vi "Initialise.vi"(8 "error in (no error)":errorcluster, 11 "Max Steps (100)":i32=3) -> (0 "error out":errorcluster, 3 "Sequencer out":refnum<class "Sequencer.lvclass">)   [LabVIEW 2015, in "Sequencer.lvclass"]
uses:
  Sequencer.lvclass
  Single Step Data.ctl
  Messaging/Message/Message.lvclass
  Sequencer.lvclass/Sequencer.ctl
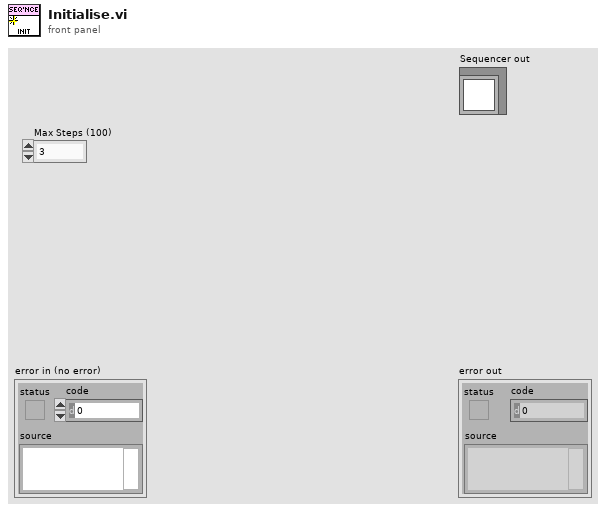
[diagram p1: front panel]
types:
  T1 = typedef "Sequencer.lvclass/Single Step Data.ctl" = cluster{"Step":string, "Parameter":variant, "Reply Channel":refnum<notifier>}
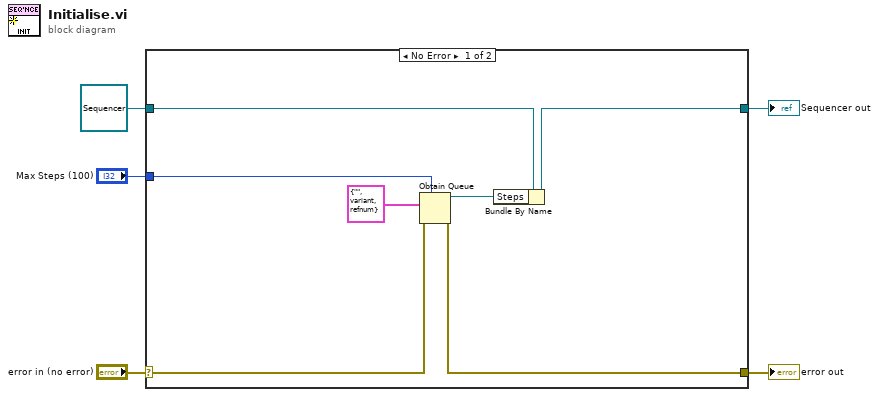
[diagram p0: block diagram]
diagram:
  n1 = case shown="No Error" "error in (no error)" {
    selector: "error in (no error)" -> [w7 w14]
    tunnel: [w6 w14] -> w4
    tunnel: [w8 w13] -> w2
    tunnel: refnum<class "Sequencer.lvclass"> refnum ("Sequencer in") -> [w10 w13]
    tunnel: "Max Steps (100)" -> [w11 _]
    frame No Error {
      n2 = Obtain Queue(max queue size (-1, unlimited)=w11, element data type=T1 {"Step"="", "Parameter"=variant, "Reply Channel"=refnum} ("Cluster"), error in (no error)=w7) -> (queue out=w9:refnum<queue>, error out=w6:errorcluster)  [unwired: 2 in, 1 out]
      n3 = Bundle By Name(cluster=w10, "Steps"=w9) -> (w8:refnum<class "Sequencer.lvclass">)
    }
    frame Error {
    }
  }
  "error out" <- w4
  "Sequencer out" <- w2
